vi "TCP-String Response.vi"(0 "connection ID":refnum<k5>, 7 "string":string="OK", 11 "error in (no error)":errorcluster) -> (4 "connection ID out":refnum<k5>, 15 "error out":errorcluster)   [LabVIEW 2020]
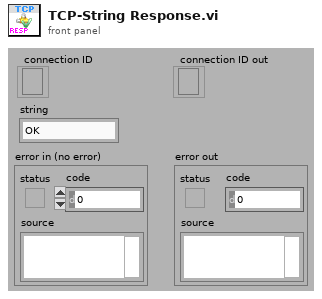
[diagram p1: front panel]
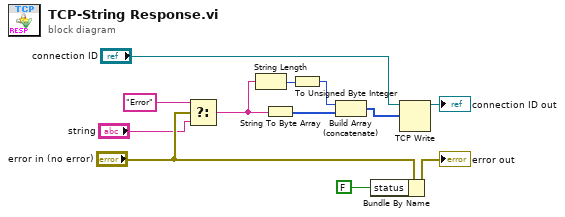
[diagram p0: block diagram]
diagram:
  n1 = Select(t="Error", s="error in (no error)", f="string") -> (s? t:f=w3:string)
  n2 = String Length(string=w3) -> (length=w6:i32)
  n3 = String To Byte Array(string=w3) -> (unsigned byte array=w8:u8[])
  n4 = To Unsigned Byte Integer(number=w6) -> (unsigned 8bit integer=w5:u8)
  n5 = Build Array (concatenate)(w5, w8) -> (w7:u8[])
  n6 = Bundle By Name(cluster="error in (no error)", "status"=FALSE) -> (→"error out":errorcluster)
  n7 = TCP Write(connection ID="connection ID", data in=w7) -> (connection ID out=→"connection ID out":refnum<k5>)  [unwired: 2 in, 2 out]
